vi "Create Client.vi"(8 "error in":errorcluster, 10 "Server Certificate File (.crt)":path, 11 "address":string) -> (0 "error out":errorcluster, 3 "gRPC ID Out":T1)   [LabVIEW 2021, in "CIFCoreWrapper.lvlib"]
uses:
  CIFCoreWrapper.lvlib
  <vilib>/gRPC/LabVIEW gRPC Library/Shared/grpcId.ctl
  <vilib>/gRPC/LabVIEW gRPC Library/grpc-lvsupport-release.lvlib
  CIFCorePlugin_client/CIFCorePlugin_client.lvlib
  CIFCoreChannel_client/CIFCoreChannel_client.lvlib
  CIFUtilities/CIFConfigurationFile/CIF Configuration File.lvlib
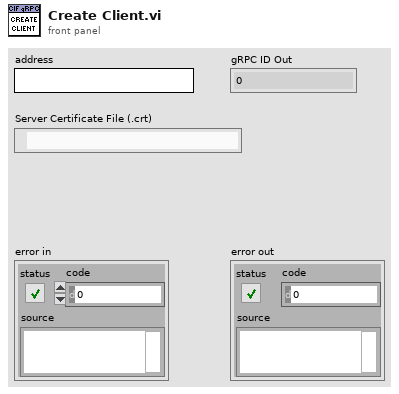
[diagram p1: front panel]
types:
  T1 = typedef "grpc-lvsupport-release.lvlib/grpcId.ctl" = u64
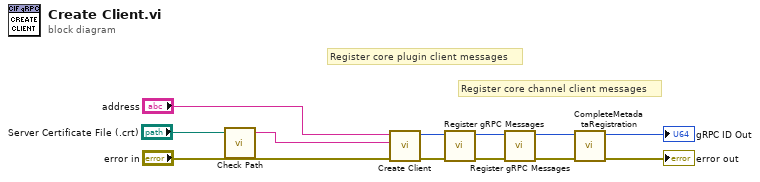
[diagram p0: block diagram]
diagram:
  # "Register core channel client messages"
  # "Register core plugin client messages"
  n1 = call "Check Path.vi"("path"="Server Certificate File (.crt)") -> ("Path String"=w1:string)  [unwired: 3 in]
  n2 = call <vilib>:"Create Client.vi"("error in"="error in", "certificatePath"=w1, "address"="address") -> ("error out"=w7:errorcluster, "ClientID out"=w8:T1)  [unwired: 7 in]
  n3 = call "Register gRPC Messages.vi"("error in (no error)"=w7, "gRPC ID"=w8) -> ("error out"=w6:errorcluster, "gRPC ID Out"=w3:T1)  [unwired: 8 in]
  n4 = call "Register gRPC Messages.vi"("error in (no error)"=w6, "gRPC ID"=w3) -> ("error out"=w5:errorcluster, "gRPC ID Out"=w4:T1)  [unwired: 8 in]
  n5 = call <vilib>:"CompleteMetadataRegistration.vi"("error in"=w5, "gRPC ID in"=w4) -> ("error out"=→"error out":errorcluster, "gRPC ID Out"=→"gRPC ID Out":T1)  [unwired: 8 in]
